vi "getParameters.vi"(11 "ExitCommand in":refnum<class "ExitCommand.lvclass">) -> (2 "Parameters":T1, 3 "ExitCommand out":refnum<class "ExitCommand.lvclass">)   [LabVIEW 2016, in "ExitCommand.lvclass"]
uses:
  ExitCommand.lvclass
  DataTypes/Topics/CommandExit.ctl
  DataTypes/Topics/Parts/CommandId.ctl
  ExitCommand.lvclass/ExitCommand.ctl
  DataTypes/Topics/M1M3SupportTopics.lvlib
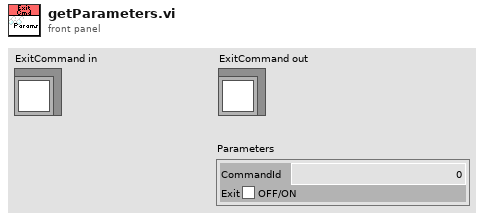
[diagram p1: front panel]
types:
  T1 = typedef "M1M3SupportTopics.lvlib/CommandExit.ctl" = cluster{"CommandId":T2, "Exit":bool}
  T2 = typedef "M1M3SupportTopics.lvlib/CommandId.ctl" = i32
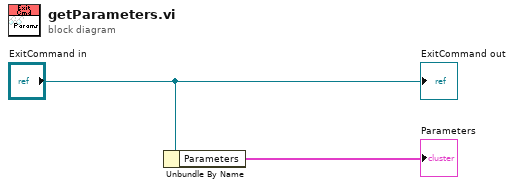
[diagram p0: block diagram]
diagram:
  n1 = Unbundle By Name("ExitCommand in") -> ("Parameters"=→"Parameters":T1)
  "ExitCommand out" <- "ExitCommand in"
